vi "SFC_Collect Re Work.vi"(5 "UserNo":string, 6 "CURSTS":string, 7 "PO":string, 8 "error in (no error)":errorcluster caption="错误输入（无错误）", 9 "MODEL":string, 10 "SID":string, 11 "Traceability 引用句柄":refnum<k24>) -> (0 "error out":errorcluster caption="错误输出", 2 "SFC_CollectReWorkSN":string, 3 "Traceability 引用句柄输出":refnum<k24>)   [LabVIEW 2014, in "Traceability.lvlib"]
uses:
  D:/webservice/Traceability.dll
  Traceability.dll
  Traceability.lvlib
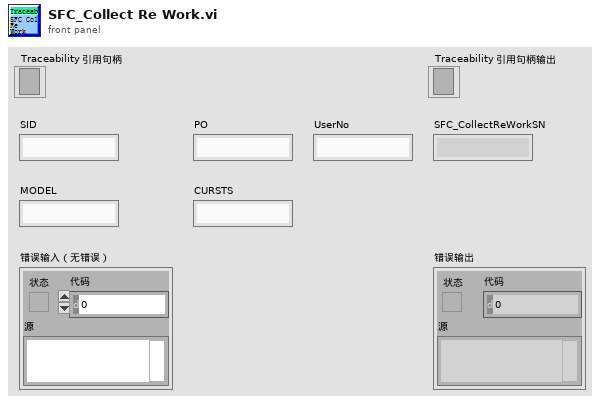
[diagram p1: front panel]
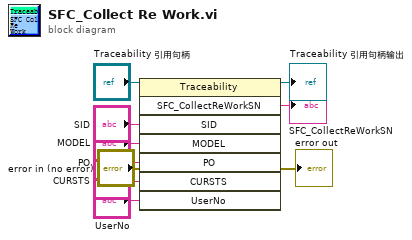
[diagram p0: block diagram]
diagram:
  n1 = invoke class="Traceability" method="SFC_CollectReWorkSN"(reference="Traceability 引用句柄", error in="error in (no error)", "SID"="SID", "MODEL"="MODEL", "PO"="PO", "CURSTS"="CURSTS", "UserNo"="UserNo") -> (reference out=→"Traceability 引用句柄输出":refnum<k24>, error out=→"error out":errorcluster, "SFC_CollectReWorkSN"=→"SFC_CollectReWorkSN":string)  [unwired: 1 in, 5 out]
